vi "UTF-8 to Text.vi"   [LabVIEW 2020, in "G-Unicode.lvlib"]
uses:
  G-Unicode.lvlib
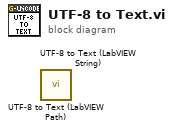
[diagram p0: block diagram]
diagram:
  n1 = call "UTF-8 to Text (LabVIEW Path).vi"() -> ()  [unwired: 10 in, 2 out]
  n2 = call "UTF-8 to Text (LabVIEW String).vi"() -> ()  [unwired: 10 in, 2 out]
